vi "Playback Audio (Polymorphic Template).vi"   [LabVIEW 2020]
uses:
  51db628f-b416-4f8e-ab2e-636034692c81.vi
  0fa3bd93-8119-4c9c-814b-37bd76b17324.vi
  c53a9200-0587-42e9-85b9-00ec2433d4a6.vi
  de2a6ab2-58a2-430e-922b-075ee1116dd1.vi
  79431ed8-0937-495f-b816-ef16c96f518d.vi
  a5a9878f-0c90-40a1-9ad5-1a9c4fe369ac.vi
  2d5ea3a0-38af-4329-b3c4-c67808aab7c9.vi
  8bb60233-bc6e-482c-9721-d4a10054c3dd.vi
  bccb6d69-3022-4ea1-8e2d-add5c581d4d5.vi
  4eac8c03-658c-404d-b9b5-b4fae04f42b4.vi
  eda577a4-4db5-441f-9df7-96d476ab2c22.vi
  fe199b84-74ad-4b8a-a31a-a7aa29bb7ecf.vi
  9404ffcd-12f7-4e0d-97c4-698e41902c53.vi
  86ef2af3-0bc5-4651-ad73-daa90fbae2f1.vi
  d91ddfc0-6d5c-4c29-b07f-934d46fadf58.vi
  f76cf793-c9d7-4762-b504-77042d8f19d4.vi
  5a99d10b-f414-41f3-a206-042854f90bae.vi
  e9b3661f-29ff-40d0-a9f7-85637f234b63.vi
  18e30697-8a31-40cb-8460-e8734a47d232.vi
  25515d5e-0426-4a54-aa54-4b351a373491.vi
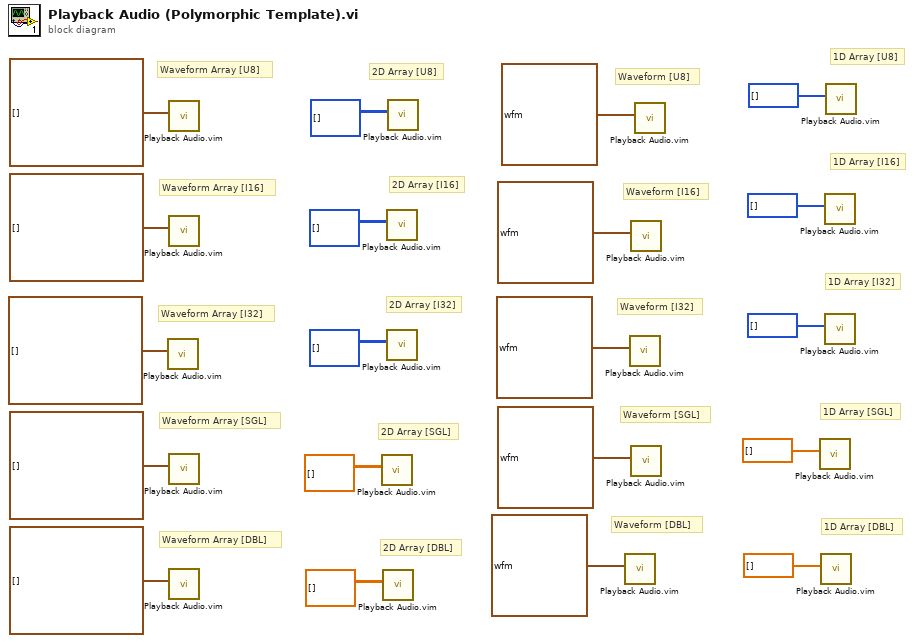
[diagram p0: block diagram]
diagram:
  # "1D Array [DBL]"
  # "1D Array [SGL]"
  # "1D Array [I32]"
  # "1D Array [I16]"
  # "1D Array [U8]"
  # "Waveform [DBL]"
  # "Waveform [SGL]"
  # "Waveform [I32]"
  # "Waveform [I16]"
  # "Waveform [U8]"
  # "2D Array [DBL]"
  # "2D Array [SGL]"
  # "2D Array [I32]"
  # "2D Array [I16]"
  # "2D Array [U8]"
  # "Waveform Array [DBL]"
  # "Waveform Array [SGL]"
  # "Waveform Array [I32]"
  # "Waveform Array [I16]"
  # "Waveform Array [U8]"
  n1 = call "Playback Audio.vim"("Audio Data"=waveform(i32)[] [] ("Data Format (I16 Waveform Array)")) -> ()  [unwired: 9 in, 2 out]
  n2 = call "Playback Audio.vim"("Audio Data"=waveform(u8)[] [] ("Data Format (I16 Waveform Array)")) -> ()  [unwired: 9 in, 2 out]
  n3 = call "Playback Audio.vim"("Audio Data"=waveform(i16)[] [] ("Data Format (I16 Waveform Array)")) -> ()  [unwired: 9 in, 2 out]
  n4 = call "Playback Audio.vim"("Audio Data"=waveform(sgl)[] [] ("Data Format (I16 Waveform Array)")) -> ()  [unwired: 9 in, 2 out]
  n5 = call "Playback Audio.vim"("Audio Data"=waveform(dbl)[] [] ("Data Format (I16 Waveform Array)")) -> ()  [unwired: 9 in, 2 out]
  n6 = call "Playback Audio.vim"("Audio Data"=sgl[][] []) -> ()  [unwired: 9 in, 2 out]
  n7 = call "Playback Audio.vim"("Audio Data"=dbl[][] []) -> ()  [unwired: 9 in, 2 out]
  n8 = call "Playback Audio.vim"("Audio Data"=i16[][] []) -> ()  [unwired: 9 in, 2 out]
  n9 = call "Playback Audio.vim"("Audio Data"=i32[][] []) -> ()  [unwired: 9 in, 2 out]
  n10 = call "Playback Audio.vim"("Audio Data"=u8[][] []) -> ()  [unwired: 9 in, 2 out]
  n11 = call "Playback Audio.vim"("Audio Data"=waveform(dbl) {"t0"=timestamp(0 s since 1904-01-01), "dt"=1.0, "Y"=[]} ("Waveform")) -> ()  [unwired: 9 in, 2 out]
  n12 = call "Playback Audio.vim"("Audio Data"=waveform(i32) {"t0"=timestamp(0 s since 1904-01-01), "dt"=1.0, "Y"=[]} ("Waveform")) -> ()  [unwired: 9 in, 2 out]
  n13 = call "Playback Audio.vim"("Audio Data"=waveform(i16) {"t0"=timestamp(0 s since 1904-01-01), "dt"=1.0, "Y"=[]} ("Waveform")) -> ()  [unwired: 9 in, 2 out]
  n14 = call "Playback Audio.vim"("Audio Data"=waveform(sgl) {"t0"=timestamp(0 s since 1904-01-01), "dt"=1.0, "Y"=[]} ("Waveform")) -> ()  [unwired: 9 in, 2 out]
  n15 = call "Playback Audio.vim"("Audio Data"=waveform(u8) {"t0"=timestamp(0 s since 1904-01-01), "dt"=1.0, "Y"=[]} ("Waveform")) -> ()  [unwired: 9 in, 2 out]
  n16 = call "Playback Audio.vim"("Audio Data"=sgl[] []) -> ()  [unwired: 9 in, 2 out]
  n17 = call "Playback Audio.vim"("Audio Data"=dbl[] []) -> ()  [unwired: 9 in, 2 out]
  n18 = call "Playback Audio.vim"("Audio Data"=i16[] []) -> ()  [unwired: 9 in, 2 out]
  n19 = call "Playback Audio.vim"("Audio Data"=i32[] []) -> ()  [unwired: 9 in, 2 out]
  n20 = call "Playback Audio.vim"("Audio Data"=u8[] []) -> ()  [unwired: 9 in, 2 out]
